vi "Check Synced Bananas.vi"(8 "error in (no error)":errorcluster, 11 "Tamer in":refnum<class "Tamer.lvclass">) -> (0 "error out":errorcluster, 1 "Propagate Banana?":bool, 2 "Internal Banana":T1, 3 "Tamer out":refnum<class "Tamer.lvclass">)   [LabVIEW 2020, in "Tamer.lvlib" / "Tamer.lvclass"]
uses:
  Tamer.lvclass
  Internatl Banana.ctl
  Run Utilities/TypeDefs/Return Code.ctl
  Tamer.lvclass/Tamer.ctl
  d93348bc-e027-4420-884e-3696d1901616.vi
  1581383c-4159-4d31-9c58-32a3b7aea81b.vi
  <vilib>/Comparison/Less/Less Functor/Less Functor.lvclass
  Run Utilities/Run Utilities.lvlib
  TALOS/TALOS_PPL.lvlibp
  TALOS/TALOS_PPL.lvlibp/Father of all uServices/Father of all uServices/Father of all uServices.lvclass
  C:/Users/aegis/Documents/CIRCUS/TALOS/TALOS_PPL.lvlibp/Father of all uServices/Father of all uServices/Father of all uServices.lvclass
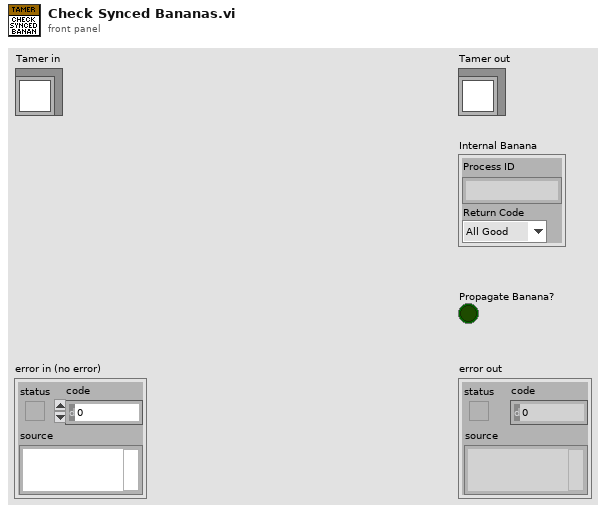
[diagram p1: front panel]
types:
  T1 = typedef "Tamer.lvlib/Tamer.lvclass/Internatl Banana.ctl" = cluster{"Process ID":string, "Return Code":T2}
  T2 = typedef "Run Utilities.lvlib/Return Code.ctl" = enum16{"All Good", "Retry", "Skip", "Skip All", "ABORT"}
  T3 = typedef "Run Utilities.lvlib/Banana Message.ctl" = cluster{"FPGA Name":string, "Return Code":T2}
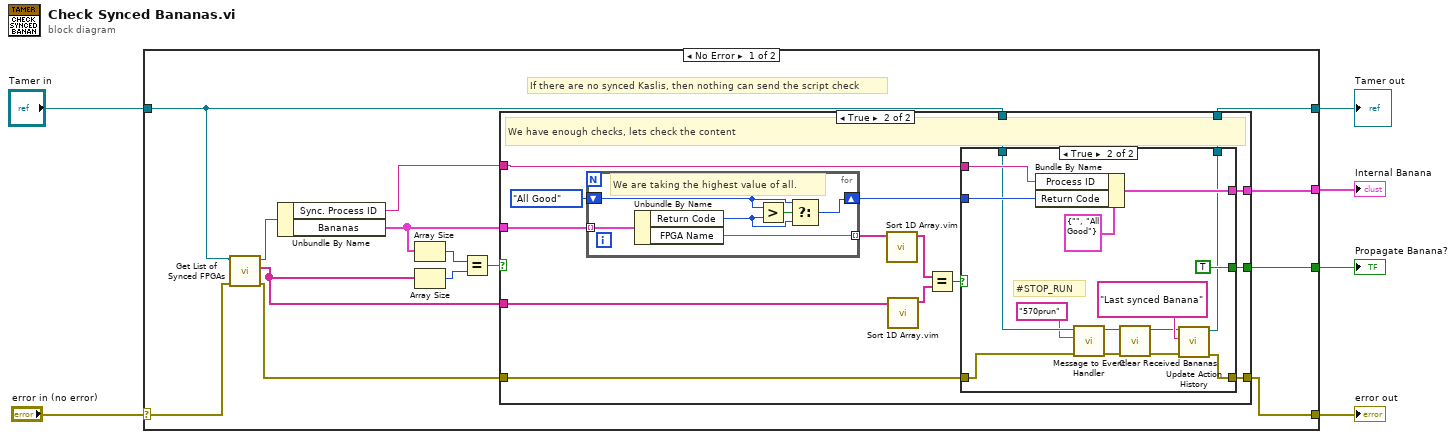
[diagram p0: block diagram]
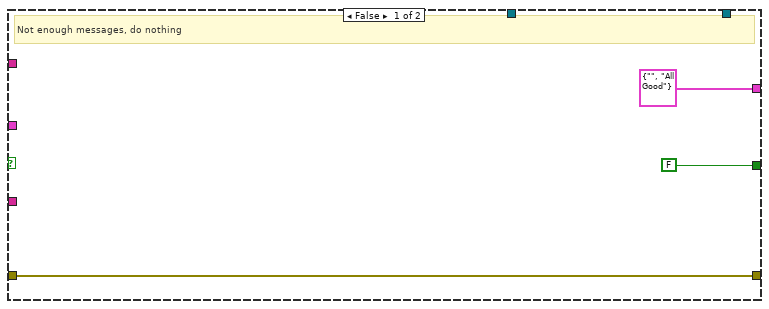
[diagram p2: hidden frame]
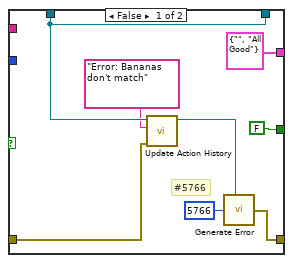
[diagram p3: hidden frame]
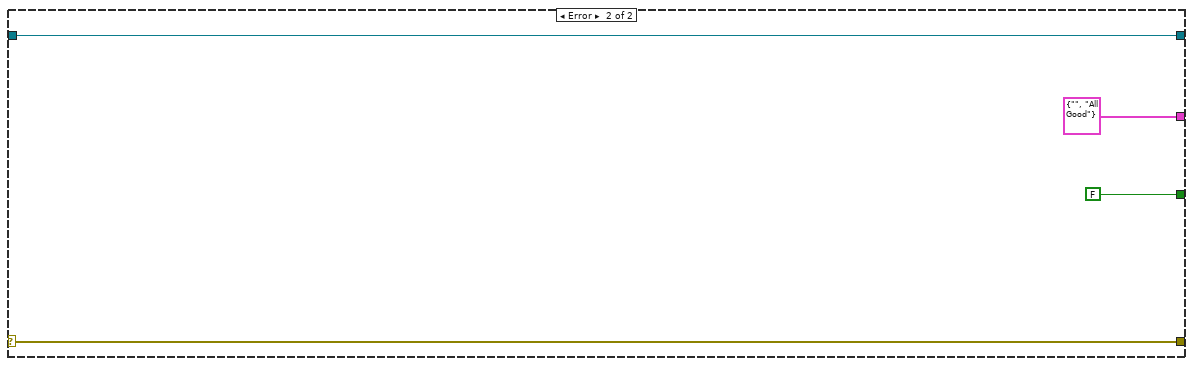
[diagram p4: hidden frame]
diagram:
  n1 = case shown="No Error" "error in (no error)" {
    selector: "error in (no error)" -> [w8 w72]
    tunnel: [w16 w72] -> w3
    tunnel: [w7 w71] -> w5
    tunnel: "Tamer in" -> [w12 w71]
    tunnel: [w14 T1 {"Process ID"="", "Return Code"=enum."All Good"} ("Internal Banana")] -> w1
    tunnel: [w13 FALSE] -> w2
    frame No Error {
      # "If there are no synced Kaslis, then nothing can send the script check"
      n2 = call-dynamic "Get List of Synced FPGAs.vi"("error in (no error)"=w8, "Tamer in"=w12) -> ("error out"=w10:errorcluster, "Synced FPGAs"=w9:string[], "Tamer out"=w11:refnum<class "Tamer.lvclass">)  [unwired: 7 in]
      n3 = Unbundle By Name(w11) -> ("Sync. Process ID"=w15:string, "Bananas"=w17:T3[])
      n4 = Array Size(array=w17) -> (size(s)=w20:i32)
      n5 = Array Size(array=w9) -> (size(s)=w19:i32)
      n6 = Equal?(x=w20, y=w19) -> (x = y?=w18:bool)
      n7 = case shown="True" w18 {
        tunnel: w17 -> [_ w39]
        tunnel: w9 -> [_ w37]
        tunnel: w12 -> [w21 w32]
        tunnel: w10 -> [w24 w31]
        tunnel: [w24 w30] -> w16
        tunnel: w15 -> [_ w29]
        tunnel: [T1 {"Process ID"="", "Return Code"=enum."All Good"} ("Internal Banana") w27] -> w14
        tunnel: [FALSE w26] -> w13
        tunnel: [w21 w25] -> w7
        frame False {
          # "Not enough messages, do nothing"
        }
        frame True {
          # "We have enough checks, lets check the content"
          n8 = for {
            tunnel: w39 -> [w68] mode=indexing
            shift-right: [w66] -> w33
            shift-left: Return_Code."All Good" ("Return Code") -> [w64]
            tunnel: [w63] -> w38 mode=indexing
            # "We are taking the highest value of all."
            n9 = Unbundle By Name(w68) -> ("Return Code"=w65:T2, "FPGA Name"=w63:string)
            n10 = Greater?(x=w64, y=w65) -> (0:w67:bool)
            n11 = Select(t=w64, s=w67, f=w65) -> (s? t:f=w66:T2)
          }
          n12 = call "Sort 1D Array.vim"("unsorted array"=w38) -> ("sorted array"=w35:string[])  [unwired: 10 in]
          n13 = call "Sort 1D Array.vim"("unsorted array"=w37) -> ("sorted array"=w36:string[])  [unwired: 10 in]
          n14 = Equal?(x=w35, y=w36) -> (x = y?=w34:bool)
          n15 = case shown="True" w34 {
            tunnel: w33 -> [_ w60]
            tunnel: w32 -> [w43 w52]
            tunnel: w31 -> [w41 w49]
            tunnel: [w47 w56] -> w30
            tunnel: w29 -> [_ w61]
            tunnel: [T1 {"Process ID"="", "Return Code"=enum."All Good"} ("Internal Banana") w59] -> w27
            tunnel: [FALSE TRUE] -> w26
            tunnel: [w43 w57] -> w25
            frame False {
              # "#5766"
              n16 = call-dynamic "Update Action History.vi"("error in (no error)"=w41, "Action"="Error: Bananas don't match", "Tamer in"=w43) -> ("Tamer out"=w42:refnum<class "Tamer.lvclass">)  [unwired: 7 in, 1 out]
              n17 = call "Generate Error.vi"("Class"=w42, "Error Code"=5766) -> ("error out"=w47:errorcluster)  [unwired: 5 in]
            }
            frame True {
              # "#STOP_RUN"
              n18 = Bundle By Name(cluster=T1 {"Process ID"="", "Return Code"=enum."All Good"} ("Internal Banana"), "Process ID"=w61, "Return Code"=w60) -> (w59:T1)
              n19 = call "Message to Event Handler.vi"("error in (no error)"=w49, "Item Name"="570prun", "uService Template in"=w52) -> ("error out"=w50:errorcluster, "uService Template out"=w51:refnum<class "Tamer.lvclass">)  [unwired: 7 in]
              n20 = call-dynamic "Clear Received Bananas.vi"("error in (no error)"=w50, "Tamer in"=w51) -> ("error out"=w53:errorcluster, "Tamer out"=w54:refnum<class "Tamer.lvclass">)  [unwired: 8 in]
              n21 = call-dynamic "Update Action History.vi"("error in (no error)"=w53, "Action"="Last synced Banana", "Tamer in"=w54) -> ("error out"=w56:errorcluster, "Tamer out"=w57:refnum<class "Tamer.lvclass">)  [unwired: 7 in]
            }
          }
        }
      }
    }
    frame Error {
    }
  }
  "error out" <- w3
  "Tamer out" <- w5
  "Propagate Banana?" <- w2
  "Internal Banana" <- w1
